vi "Timestamp String to LV Timestamp.vi"(0 "Timestamp String":string) -> (1 "Y M D H M S Array":i32[](array[numeric]), 2 "Timestamp":timestamp)   [LabVIEW 2018]
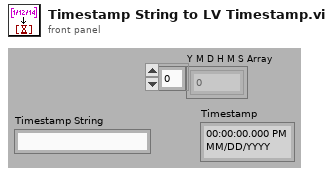
[diagram p1: front panel]
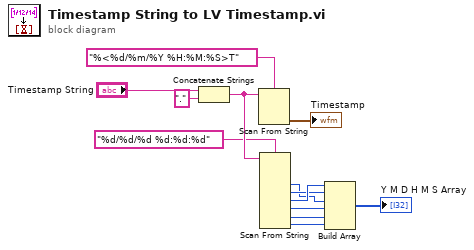
[diagram p0: block diagram]
diagram:
  n1 = Concatenate Strings("Timestamp String", "." ("string")) -> (w9:string)
  n2 = Scan From String(format string="%<%d/%m/%Y %H:%M:%S>T", input string=w9) -> (output 1=→"Timestamp":timestamp)  [unwired: 3 in, 3 out]
  n3 = Scan From String(format string="%d/%d/%d %d:%d:%d", input string=w9) -> (output 1=w5:i32, output 2=w6:i32, output 3=w7:i32, output 4=w4:i32, output 5=w3:i32, output 6=w2:i32)  [unwired: 8 in, 3 out]
  n4 = Build Array(w7, w6, w5, w4, w3, w2) -> (→"Y M D H M S Array":i32[])
